vi "Integrator Training FPGA MyRIO.vi"() -> ()   [LabVIEW 2018]
uses:
  <vilib>/Platform/TimedLoop/XDataNode/timing_clust.ctl
  <vilib>/Platform/TimedLoop/XDataNode/nitl_modes.ctl
  <vilib>/Platform/TimedLoop/XDataNode/wakeup.ctl
  <vilib>/rvi/Emulation/niFpgaGetClockAttributes.vi
  <vilib>/rvi/Emulation/niFpgaSctlEmulationGetInTimedLoop.vi
  <vilib>/rvi/Emulation/niFpgaEmulationReportErrorSimple.vi
  <vilib>/rvi/Emulation/niFpgaProcessEmulError.vi
  <vilib>/rvi/eio/common/nirviEmuTemplateMethod_errors.vi
  <vilib>/rvi/Emulation/niFpgaCriticalErrorInLSC.vi
  <vilib>/eio/EIONode/EIONode.xnode
  <vilib>/Platform/TimedLoop/XDataNode/XDataNode.xnode
  <vilib>/Platform/TimedLoop/XDataNode/XDNodeRunTimeDep.lvlib
  <vilib>/NI Veristand/FPGA/NI_VS FPGA Support.lvlib
  <userlib>/_NI VeriStand FPGA Support/NI VeriStand FPGA Clock Support/NI_VS FPGA Clock Support.lvlib
panel:
  out "from FIFO":u64[](array[numeric])
  out "to FIFO":u64[](array[numeric])
  in  "Count(Ticks)":u32
  out "Sine Out":i16
  in  "Phase offset (periods)":fxp<+,32,0>
  in  "Frequency (periods/tick)":fxp<+,32,0>=0.0002500000409781933
  in  "Generate IRQ":bool
  in  "Use External Timing":bool
  in  "Write to  RTSI":bool
  in  "Loop Rate (usec)":u32
  in  "Start":bool
  # "PWM"
  # "Configuration"
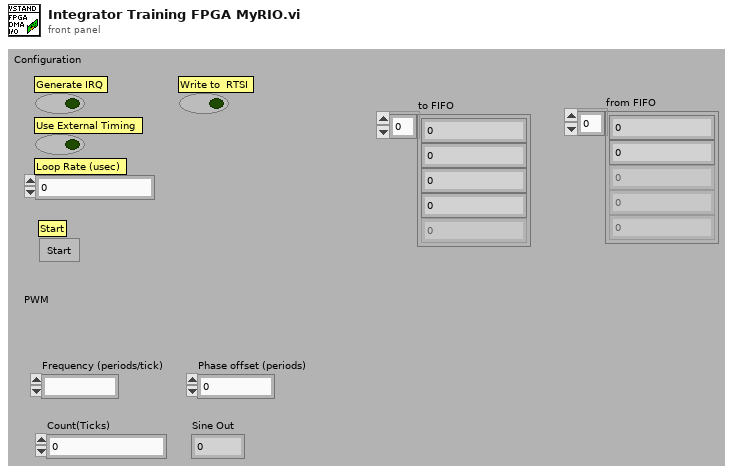
[diagram p1: front panel]
types:
  T1 = typedef "XDNodeRunTimeDep.lvlib/timing_clust.ctl" = cluster{"Expected End [f-1]":u64, "Actual End [f-1]":u64, "Finished Late? [f-1]":bool, "Expected End [i-1]":u64, "Actual End [i-1]":u64, "Finished Late? [i-1]":bool, "Expected Start [i]":u64, "Actual Start [i]":u64, "Expected Start [f]":u64, "Actual Start [f]":u64, "Source Name":string, "Structure Name":string, "Period":i64, "Deadline":i64, "Offset":i64, "Start":i64, "Priority":i32, "Timeout":i32, "Mode":T2, "Wakeup Reason":T3, "Error":errorcluster, "Source Type":string, "Secondary Source Type":string, "Global End Time":u64, "Global Start Time":u64, "Frame Duration":u64, "Iteration Duration":u64, "Assigned CPU":i32, "I/O Scan Engine Mode":u32}
  T2 = typedef "XDNodeRunTimeDep.lvlib/nitl_modes.ctl" = enum32{"No Change", "Process missed periods, maintain original phase", "Discard missed periods, maintain original phase", "Process missed periods, ignore original phase", "Discard missed periods, ignore original phase"}
  T3 = typedef "XDNodeRunTimeDep.lvlib/wakeup.ctl" = enum32{"Normal", "Aborted", "Asynchronous wakeup", "Timing source error", "Timed loop error", "Timeout"}
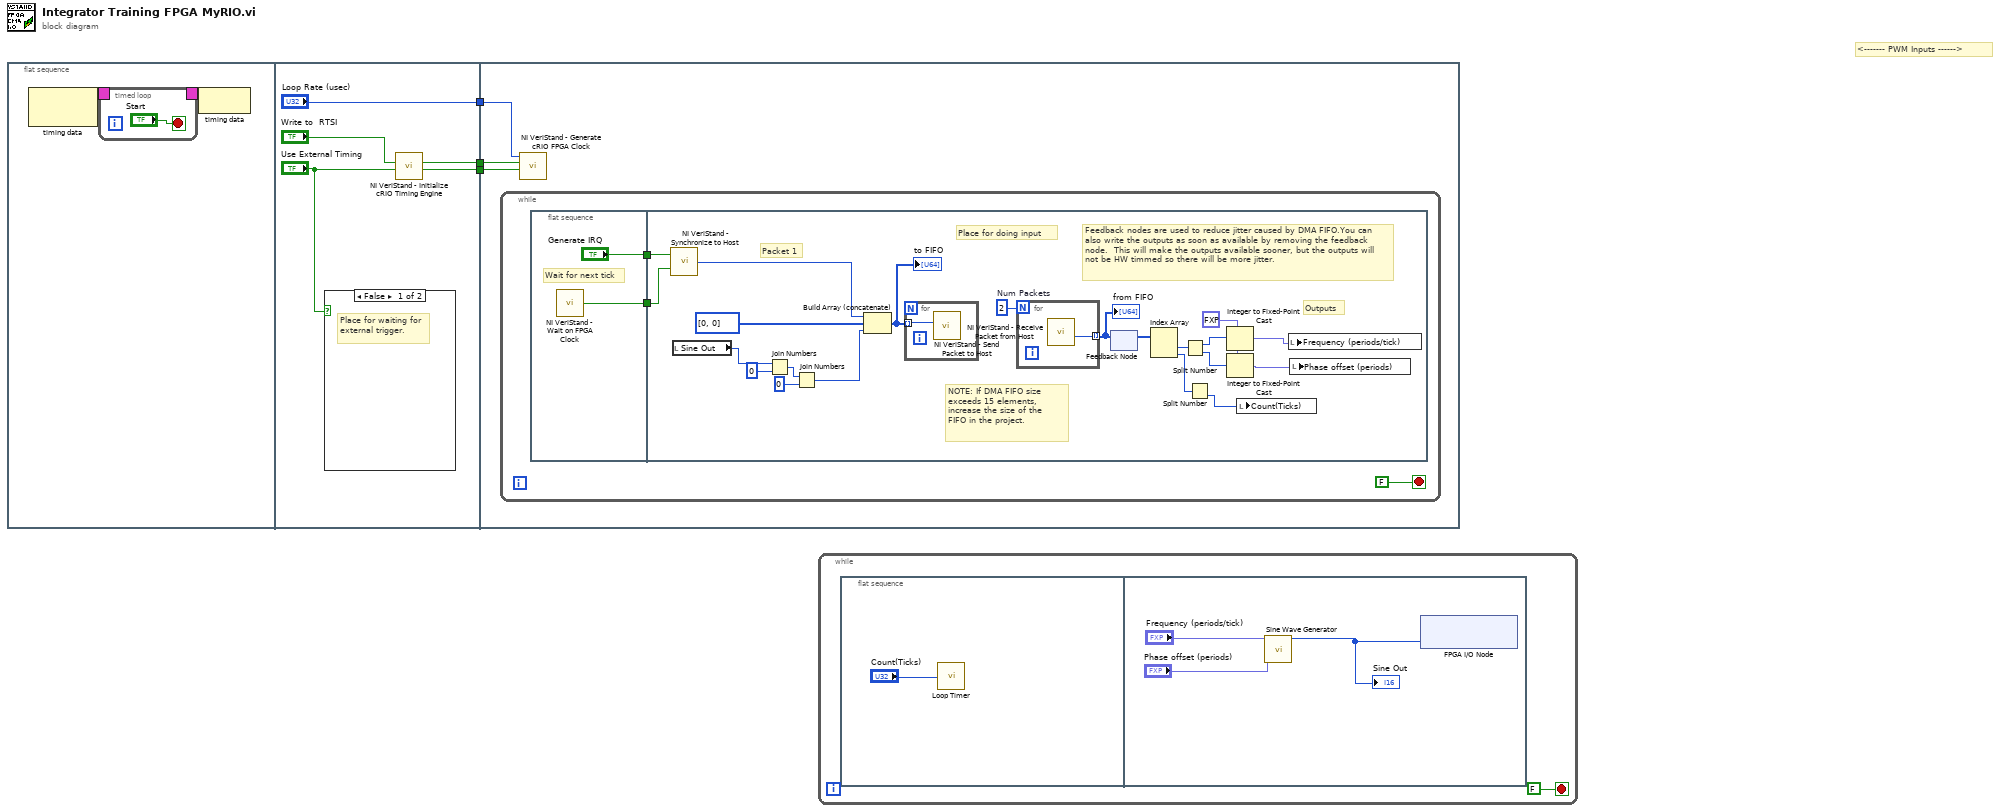
[diagram p0: block diagram]
diagram:
  # "<------- PWM Inputs ------>"
  n1 = flat-sequence {
    tunnel: [w12] -> w3
    tunnel: ["Loop Rate (usec)"] -> w2
    tunnel: [w11] -> w1
    tunnel: w3 -> [w18]
    tunnel: w2 -> [w17]
    tunnel: w1 -> [w16]
    frame #0 {
      n2 = node-c288() -> (w5:T1)  [unwired: 1 out]
      n3 = timed-loop {
        timing: w5 -> [_]
        timing-out: [_] -> w4
        stop <- "Start" stop-if-true
      }
      n4 = node-c288(w4) -> ()
    }
    frame #1 {
      n5 = case shown="False" "Use External Timing" {
        frame False {
          # "Place for waiting for external trigger."
        }
        frame True {
          # "Do not wait on trigger when externally timed."
        }
      }
      n6 = call <userlib>:"NI VeriStand - Initialize cRIO Timing Engine.vi"("Use External Timing In"="Use External Timing", "Write to  RTSI In"="Write to  RTSI") -> ("Use External Timing Out"=w12:bool, "Write to  RTSI Out"=w11:bool)  [unwired: 8 in]
    }
    frame #2 {
      n7 = while {
        stop <- FALSE stop-if-true
        n8 = flat-sequence {
          tunnel: ["Generate IRQ"] -> w20
          tunnel: [w22] -> w19
          tunnel: w20 -> [w44]
          tunnel: w19 -> [w43]
          frame #0 {
            # "Wait for next tick"
            n9 = call <userlib>:"NI VeriStand - Wait on FPGA Clock.vi"() -> ("Clock Ticked"=w22:bool)
          }
          frame #1 {
            w29 = fxp<+,32,0> 0.0 ("fixed-point type")
            w42 = 2  # Num Packets
            # "Packet 1"
            # "Outputs"
            # "NOTE: If DMA FIFO size exceeds 15 elements, increase the size of the FIFO in the project."
            # "Feedback nodes are used to reduce jitter caused by DMA FIFO.You can also write the outputs as soon as available by removing the feedback node.  This will make the outputs available sooner, but the outputs will not be HW timmed so there will be more jitter."
            # "Place for doing input"
            n10 = call <userlib>:"NI VeriStand - Synchronize to Host.vi"("Clock Ticked"=w43, "Generate IRQ"=w44) -> ("Is Late?"=w41:u64)
            n11 = local read "Sine Out"() -> (w37:i16)
            n12 = Join Numbers(hi=w37, lo=i16 0) -> ((hi.lo)=w35:u32)
            n13 = Join Numbers(hi=w35, lo=u32 0) -> ((hi.lo)=w33:u64)
            n14 = Build Array (concatenate)(w41, u64[] [0, 0] ("Packets"), w33) -> (w40:u64[])
            "to FIFO" <- w40
            n15 = for {
              tunnel: w40 -> [w45] mode=indexing
              n16 = call <vilib>:"NI VeriStand - Send Packet to Host.vi"("Element"=w45) -> ()  [unwired: 2 in, 9 out]
            }
            n17 = for {
              N: w42 -> [_]
              tunnel: [w46] -> w24 mode=indexing
              n18 = call <vilib>:"NI VeriStand - Receive Packet from Host.vi"() -> ("Element"=w46:u64)  [unwired: 2 in, 9 out]
            }
            "from FIFO" <- w24
            n19 = feedback-in #1(w24) -> ()
            n20 = feedback #1() -> (w39:u64[])  [unwired: 1 in]
            n21 = Index Array(array=w39) -> (element #1=w38:u64, element #2=w27:u64)  [unwired: 2 in]
            n22 = Split Number(x=w38) -> (hi(x)=w32:u32, lo(x)=w30:u32)
            n23 = Split Number(x=w27) -> (lo(x)=w26:u32)  [unwired: 1 out]
            n24 = Integer to Fixed-Point Cast(fixed-point type=w29, integer=w32) -> (fixed-point=w31:fxp<+,32,0>)
            n25 = Integer to Fixed-Point Cast(fixed-point type=w29, integer=w30) -> (fixed-point=w28:fxp<+,32,0>)
            n26 = local write "Count(Ticks)"(w26) -> ()
            n27 = local write "Frequency (periods/tick)"(w31) -> ()
            n28 = local write "Phase offset (periods)"(w28) -> ()
          }
        }
      }
      n29 = call <userlib>:"NI VeriStand - Generate cRIO FPGA Clock.vi"("Use External Timing"=w18, "Write to  RTSI"=w16, "Loop Rate (usec)"=w17) -> ()  [unwired: 9 in]
    }
  }
  n30 = while {
    stop <- FALSE stop-if-true
    n31 = flat-sequence {
      frame #0 {
        n32 = call "Loop Timer"("Count(Ticks)"="Count(Ticks)") -> ()  [unwired: 1 out]
      }
      frame #1 {
        n33 = call "Sine Wave Generator"("frequency (periods/tick)"="Frequency (periods/tick)", "phase offset (periods)"="Phase offset (periods)") -> ("sine out"=w49:i16)  [unwired: 13 in]
        "Sine Out" <- w49
        n34 = xnode "FPGA I/O Node"("NI 9262/AO0"=w49) -> ()  [unwired: 1 in, 1 out]
      }
    }
  }
